vi "PID_controller_05.vi"() -> ()   [LabVIEW 2011]
uses:
  <vilib>/Platform/TimedLoop/XDataNode/nitl_modes.ctl
  <vilib>/Platform/TimedLoop/XDataNode/timing_clust.ctl
  <vilib>/Platform/TimedLoop/XDataNode/wakeup.ctl
  <vilib>/Platform/TimedLoop/XDataNode/XDataNode.xnode
  <vilib>/Platform/TimedLoop/XDataNode/XDNodeRunTimeDep.lvlib
panel:
  out "Numeric":dbl
  out "x-y":dbl
  out "S00":dbl
  out "S10":dbl
  out "S20":dbl
  out "S11":dbl
  out "S01":dbl
  out "weight":dbl[](array[numeric])
  in  "# of points to watch":i32
  in  "alpha":dbl=-1.0
  out "t0":dbl
  out "error(t)":cluster{dbl, "Value":dbl}[](array[cluster])
  out "error out":errorcluster
  out "first":bool=TRUE
  out "P (torr)":string
  out "XY Graph":cluster{dbl, "Value":dbl}[](graph)
  out "current value":dbl
  in  "stop":bool
  in  "Period (s)":dbl
  out "dValue":dbl
  out "derivative":dbl
  out "integral":dbl
  out "error":dbl
  out "Current angle (deg)":dbl
  in  "Kd":dbl
  in  "Ki":dbl
  in  "Kp":dbl
  out "Current P (torr)":dbl
  in  "Set Point (torr)":dbl
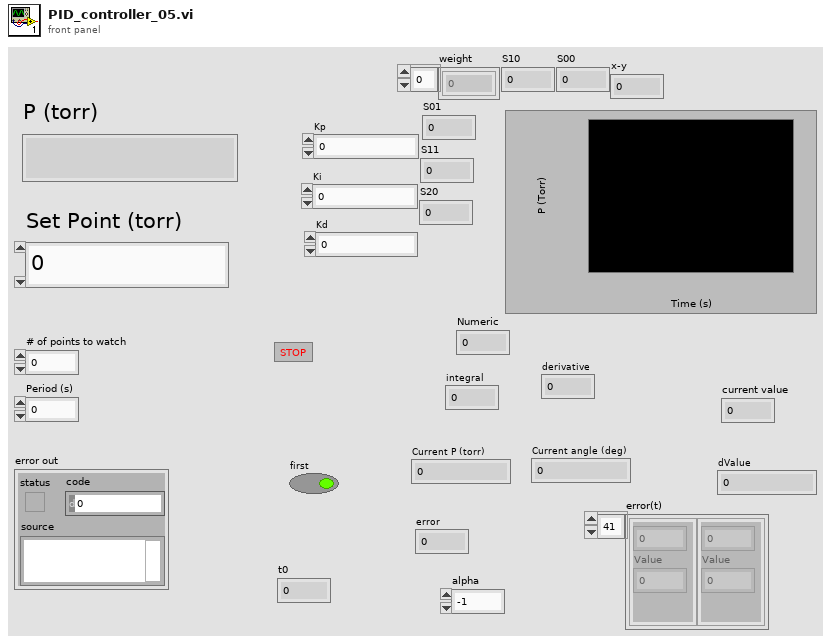
[diagram p1: front panel]
types:
  T1 = typedef "XDNodeRunTimeDep.lvlib/nitl_modes.ctl" = enum32{"No Change", "Process missed periods, maintain original phase", "Discard missed periods, maintain original phase", "Process missed periods, ignore original phase", "Discard missed periods, ignore original phase"}
  T2 = typedef "XDNodeRunTimeDep.lvlib/timing_clust.ctl" = cluster{"Expected End [f-1]":u64, "Actual End [f-1]":u64, "Finished Late? [f-1]":bool, "Expected End [i-1]":u64, "Actual End [i-1]":u64, "Finished Late? [i-1]":bool, "Expected Start [i]":u64, "Actual Start [i]":u64, "Expected Start [f]":u64, "Actual Start [f]":u64, "Source Name":string, "Structure Name":string, "Period":i64, "Deadline":i64, "Offset":i64, "Start":i64, "Priority":i32, "Timeout":i32, "Mode":T1, "Wakeup Reason":T3, "Error":errorcluster, "Source Type":string, "Secondary Source Type":string, "Global End Time":u64, "Global Start Time":u64, "Frame Duration":u64, "Iteration Duration":u64, "Assigned CPU":i32, "I/O Scan Engine Mode":u32}
  T3 = typedef "XDNodeRunTimeDep.lvlib/wakeup.ctl" = enum32{"Normal", "Aborted", "Asynchronous wakeup", "Timing source error", "Timed loop error", "Timeout"}
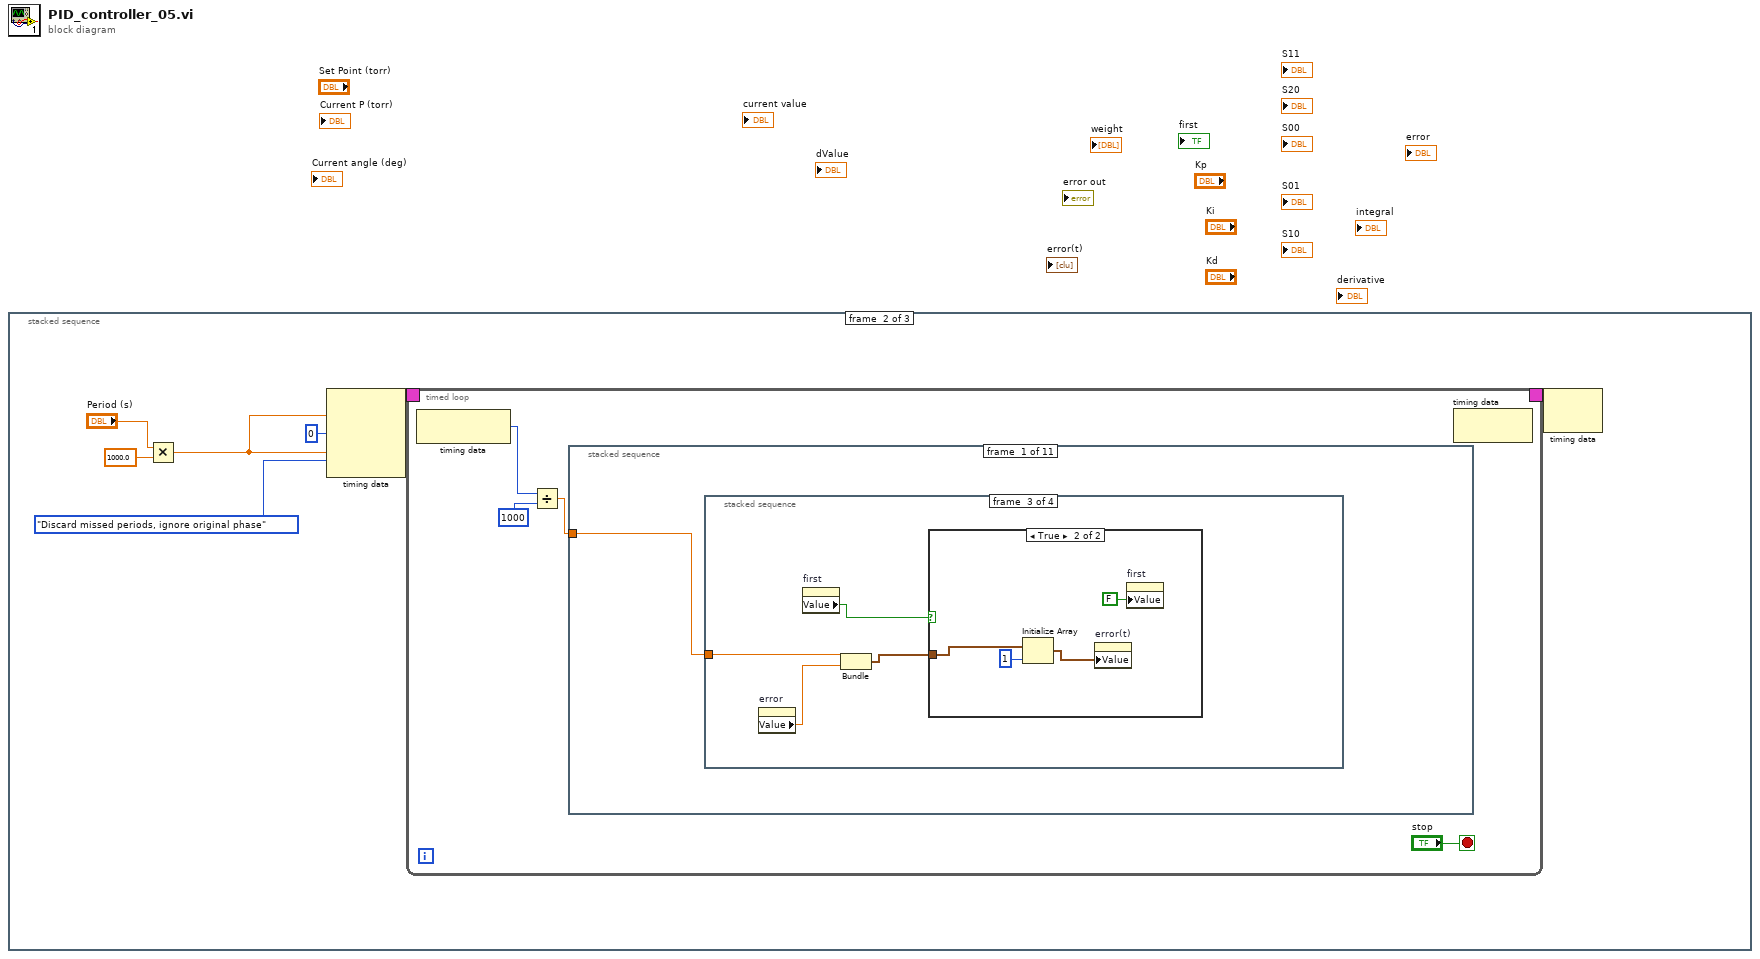
[diagram p0: block diagram]
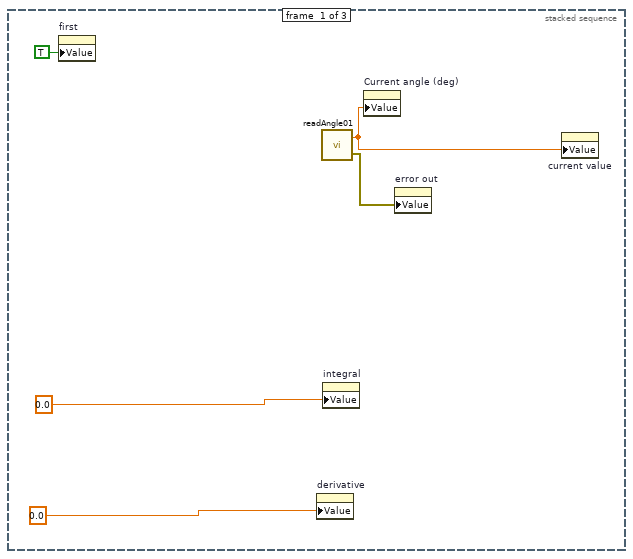
[diagram p2: hidden frame]
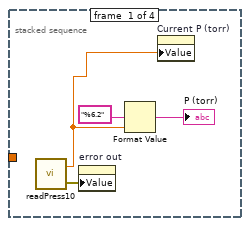
[diagram p3: hidden frame]
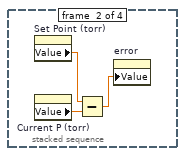
[diagram p4: hidden frame]
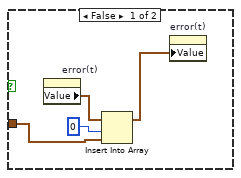
[diagram p5: hidden frame]
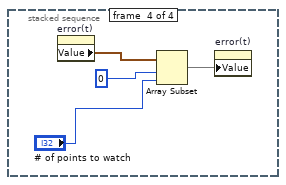
[diagram p6: hidden frame]
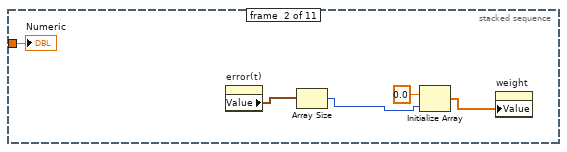
[diagram p7: hidden frame]
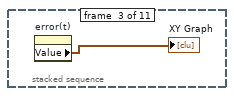
[diagram p8: hidden frame]
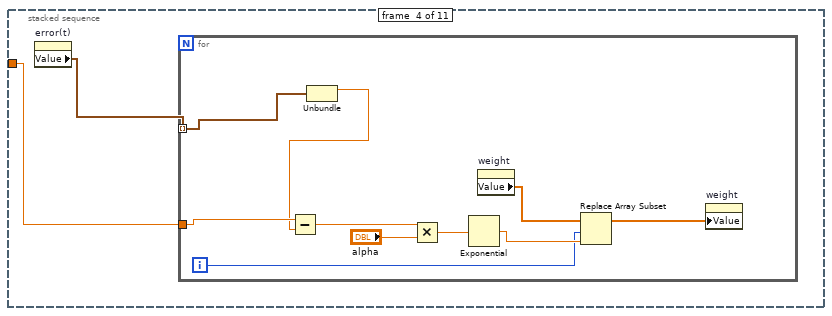
[diagram p9: hidden frame]
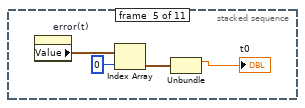
[diagram p10: hidden frame]
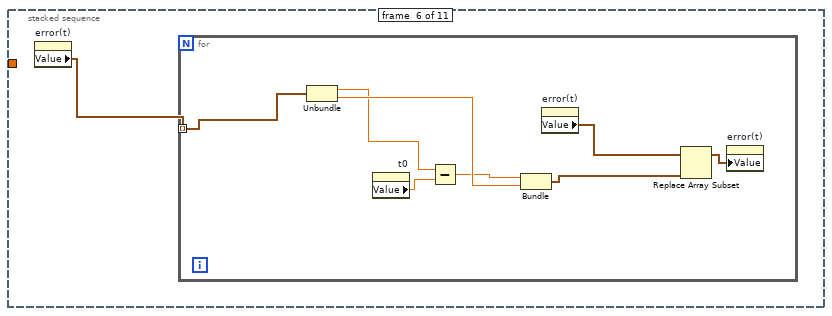
[diagram p11: hidden frame]
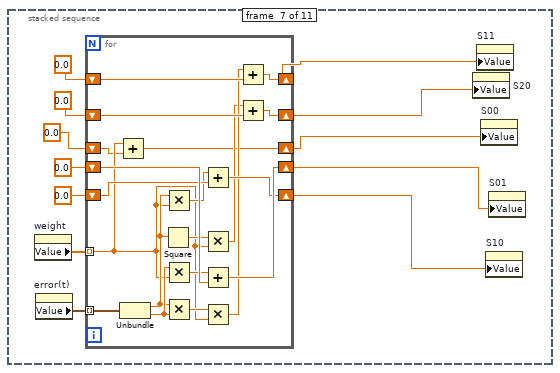
[diagram p12: hidden frame]
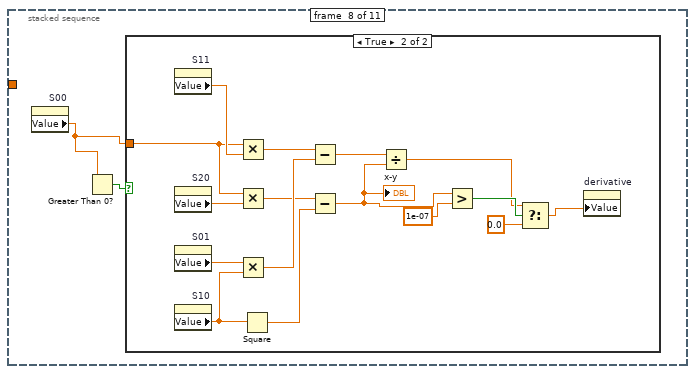
[diagram p13: hidden frame]
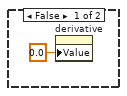
[diagram p14: hidden frame]
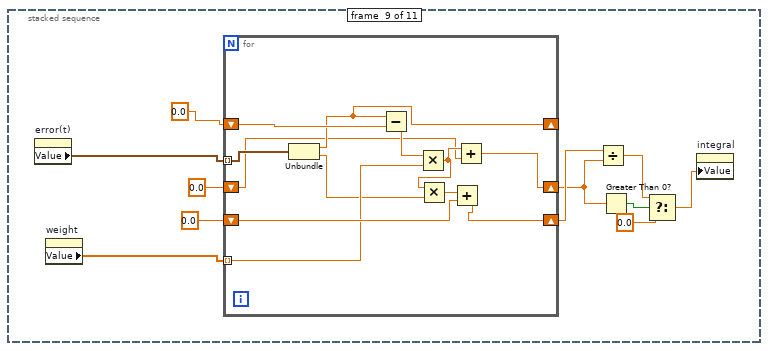
[diagram p15: hidden frame]
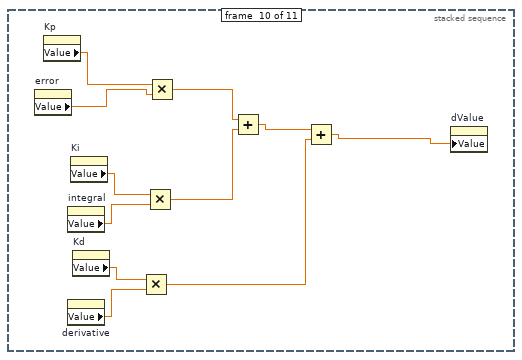
[diagram p16: hidden frame]
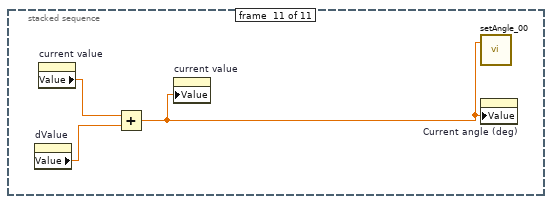
[diagram p17: hidden frame]
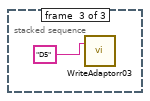
[diagram p18: hidden frame]
diagram:
  n1 = stacked-sequence {
    frame #0 {
      n2 = property on="first" class="Bool (strict)"("Value"=TRUE ("first")) -> ()  [unwired: 2 in, 2 out]
      n3 = property on="derivative" class="DigNum (strict)"("Value"=0.0 ("derivative")) -> ()  [unwired: 2 in, 2 out]
      n4 = call "readAngle01.vi"() -> ("angle"=w1:dbl, "error out"=w2:errorcluster)  [unwired: 1 in]
      n5 = property on="integral" class="DigNum (strict)"("Value"=0.0 ("integral")) -> ()  [unwired: 2 in, 2 out]
      n6 = property on="Current angle (deg)" class="DigNum (strict)"("Value"=w1) -> ()  [unwired: 2 in, 2 out]
      n7 = property on="error out" class="Clust (strict)"("Value"=w2) -> ()  [unwired: 2 in, 2 out]
      n8 = property on="current value" class="DigNum (strict)"("Value"=w1) -> ()  [unwired: 2 in, 2 out]
    }
    frame #1 {
      n9 = Multiply(x="Period (s)", y=1000.0) -> (x*y=w7:dbl)
      n10 = node-c288(w7, i64 0 ("Offset"), w7, nitl_modes."Discard missed periods, ignore original phase" ("Mode")) -> (w12:T2)
      n11 = timed-loop {
        timing: w12 -> [_]
        timing-out: [_] -> w11
        stop <- "stop" stop-if-true
        n12 = node-c288() -> (w13:i64)  [unwired: 1 in]
        n13 = Divide(x=w13, y=i64 1000) -> (x/y=w14:dbl)
        n14 = stacked-sequence {
          tunnel: w14 -> [w17 w41 _ w47 _ _ _ _ _ _ _]
          frame #0 {
            n15 = stacked-sequence {
              tunnel: w17 -> [_ _ w27 _]
              frame #0 {
                n16 = call "readPress10.vi"() -> ("P"=w18:dbl, "error out"=w19:errorcluster)  [unwired: 1 in]
                n17 = property on="error out" class="Clust (strict)"("Value"=w19) -> ()  [unwired: 2 in, 2 out]
                n18 = Format Value(format string="%6.2", value (0)=w18) -> (output string=→"P (torr)":string)  [unwired: 1 in]
                n19 = property on="Current P (torr)" class="DigNum (strict)"("Value"=w18) -> ()  [unwired: 2 in, 2 out]
              }
              frame #1 {
                n20 = property on="Set Point (torr)" class="DigNum (strict)"() -> ("Value"=w23:dbl)  [unwired: 2 in, 2 out]
                n21 = property on="Current P (torr)" class="DigNum (strict)"() -> ("Value"=w24:dbl)  [unwired: 2 in, 2 out]
                n22 = Subtract(x=w23, y=w24) -> (x-y=w22:dbl)
                n23 = property on="error" class="DigNum (strict)"("Value"=w22) -> ()  [unwired: 2 in, 2 out]
              }
              frame #2 {
                n24 = property on="error" class="DigNum (strict)"() -> ("Value"=w26:dbl)  [unwired: 2 in, 2 out]
                n25 = property on="first" class="Bool (strict)"() -> ("Value"=w28:bool)  [unwired: 2 in, 2 out]
                n26 = Bundle(w27, "Value"=w26) -> (w25:cluster{dbl, "Value":dbl})  [unwired: 1 in]
                n27 = case shown="True" w28 {
                  tunnel: w25 -> [w30 w35]
                  frame False {
                    n28 = property on="error(t)" class="Arr (strict)"() -> ("Value"=w31:cluster{dbl, "Value":dbl}[])  [unwired: 2 in, 2 out]
                    n29 = Insert Into Array(array=w31, index=0, new element=w30) -> (w29:cluster{dbl, "Value":dbl}[])
                    n30 = property on="error(t)" class="Arr (strict)"("Value"=w29) -> ()  [unwired: 2 in, 2 out]
                  }
                  frame True {
                    n31 = Initialize Array(w35, 1 ("dimension size")) -> (w33:cluster{dbl, "Value":dbl}[])
                    n32 = property on="error(t)" class="Arr (strict)"("Value"=w33) -> ()  [unwired: 2 in, 2 out]
                    n33 = property on="first" class="Bool (strict)"("Value"=FALSE ("first")) -> ()  [unwired: 2 in, 2 out]
                  }
                }
              }
              frame #3 {
                n34 = property on="error(t)" class="Arr (strict)"() -> ("Value"=w38:cluster{dbl, "Value":dbl}[])  [unwired: 2 in, 2 out]
                n35 = Array Subset(array=w38, index=0, length="# of points to watch") -> (w40:cluster{dbl, "Value":dbl}[])
                n36 = property on="error(t)" class="Arr (strict)"("Value"=w40) -> ()  [unwired: 2 in, 2 out]
              }
            }
          }
          frame #1 {
            n37 = property on="error(t)" class="Arr (strict)"() -> ("Value"=w45:cluster{dbl, "Value":dbl}[])  [unwired: 2 in, 2 out]
            n38 = Array Size(array=w45) -> (size(s)=w43:i32)
            n39 = Initialize Array(0.0 ("element"), w43) -> (w42:dbl[])
            n40 = property on="weight" class="Arr (strict)"("Value"=w42) -> ()  [unwired: 2 in, 2 out]
            "Numeric" <- w41
          }
          frame #2 {
            n41 = property on="error(t)" class="Arr (strict)"() -> ("Value"=→"XY Graph":cluster{dbl, "Value":dbl}[])  [unwired: 2 in, 2 out]
          }
          frame #3 {
            n42 = property on="error(t)" class="Arr (strict)"() -> ("Value"=w48:cluster{dbl, "Value":dbl}[])  [unwired: 2 in, 2 out]
            n43 = for {
              tunnel: w48 -> [w58] mode=indexing
              tunnel: w47 -> [w55]
              i -> [w50]
              n44 = Unbundle(w58) -> (w54:dbl)  [unwired: 1 out]
              n45 = Subtract(x=w55, y=w54) -> (x-y=w53:dbl)
              n46 = Multiply(x=w53, y="alpha") -> (x*y=w56:dbl)
              n47 = Exponential(1:w56) -> (0:w52:dbl)
              n48 = property on="weight" class="Arr (strict)"() -> ("Value"=w51:dbl[])  [unwired: 2 in, 2 out]
              n49 = Replace Array Subset(array=w51, new element=w52, index=w50) -> (w49:dbl[])
              n50 = property on="weight" class="Arr (strict)"("Value"=w49) -> ()  [unwired: 2 in, 2 out]
            }
          }
          frame #4 {
            n51 = property on="error(t)" class="Arr (strict)"() -> ("Value"=w62:cluster{dbl, "Value":dbl}[])  [unwired: 2 in, 2 out]
            n52 = Index Array(array=w62, index=0) -> (element=w60:cluster{dbl, "Value":dbl})
            n53 = Unbundle(w60) -> (→"t0":dbl)  [unwired: 1 out]
          }
          frame #5 {
            n54 = property on="error(t)" class="Arr (strict)"() -> ("Value"=w63:cluster{dbl, "Value":dbl}[])  [unwired: 2 in, 2 out]
            n55 = for {
              tunnel: w63 -> [w68] mode=indexing
              n56 = Unbundle(w68) -> (w65:dbl, "Value"=w70:dbl)
              n57 = property on="t0" class="DigNum (strict)"() -> ("Value"=w71:dbl)  [unwired: 2 in, 2 out]
              n58 = Subtract(x=w65, y=w71) -> (x-y=w66:dbl)
              n59 = Bundle(w66, "Value"=w70) -> (w64:cluster{dbl, "Value":dbl})  [unwired: 1 in]
              n60 = property on="error(t)" class="Arr (strict)"() -> ("Value"=w69:cluster{dbl, "Value":dbl}[])  [unwired: 2 in, 2 out]
              n61 = Replace Array Subset(array=w69, new element=w64) -> (w67:cluster{dbl, "Value":dbl}[])  [unwired: 1 in]
              n62 = property on="error(t)" class="Arr (strict)"("Value"=w67) -> ()  [unwired: 2 in, 2 out]
            }
          }
          frame #6 {
            n63 = property on="weight" class="Arr (strict)"() -> ("Value"=w78:dbl[])  [unwired: 2 in, 2 out]
            n64 = property on="error(t)" class="Arr (strict)"() -> ("Value"=w83:cluster{dbl, "Value":dbl}[])  [unwired: 2 in, 2 out]
            n65 = for {
              tunnel: w83 -> [w99] mode=indexing
              shift-right: [w100] -> w73
              shift-left: 0.0 -> [w103]
              shift-right: [w96] -> w76
              shift-left: 0.0 -> [w102]
              shift-right: [w95] -> w75
              shift-left: 0.0 -> [w101]
              shift-right: [w97] -> w72
              shift-left: 0.0 -> [w98]
              tunnel: w78 -> [w86] mode=indexing
              shift-right: [w84] -> w74
              shift-left: 0.0 -> [w85]
              n66 = Add(x=w86, y=w85) -> (x+y=w84:dbl)
              n67 = Unbundle(w99) -> (w88:dbl, "Value"=w94:dbl)
              n68 = Square(x=w88) -> (x^2=w90:dbl)
              n69 = Multiply(x=w88, y=w86) -> (x*y=w87:dbl)
              n70 = Multiply(x=w94, y=w86) -> (x*y=w93:dbl)
              n71 = Multiply(x=w88, y=w94) -> (x*y=w92:dbl)
              n72 = Add(x=w87, y=w98) -> (x+y=w97:dbl)
              n73 = Multiply(x=w90, y=w86) -> (x*y=w89:dbl)
              n74 = Add(x=w93, y=w103) -> (x+y=w100:dbl)
              n75 = Multiply(x=w92, y=w86) -> (x*y=w91:dbl)
              n76 = Add(x=w91, y=w102) -> (x+y=w96:dbl)
              n77 = Add(x=w89, y=w101) -> (x+y=w95:dbl)
            }
            n78 = property on="S20" class="DigNum (strict)"("Value"=w75) -> ()  [unwired: 2 in, 2 out]
            n79 = property on="S11" class="DigNum (strict)"("Value"=w76) -> ()  [unwired: 2 in, 2 out]
            n80 = property on="S00" class="DigNum (strict)"("Value"=w74) -> ()  [unwired: 2 in, 2 out]
            n81 = property on="S10" class="DigNum (strict)"("Value"=w72) -> ()  [unwired: 2 in, 2 out]
            n82 = property on="S01" class="DigNum (strict)"("Value"=w73) -> ()  [unwired: 2 in, 2 out]
          }
          frame #7 {
            n83 = property on="S00" class="DigNum (strict)"() -> ("Value"=w104:dbl)  [unwired: 2 in, 2 out]
            n84 = Greater Than 0?(x=w104) -> (x > 0?=w105:bool)
            n85 = case shown="True" w105 {
              tunnel: w104 -> [_ w114]
              frame False {
                n86 = property on="derivative" class="DigNum (strict)"("Value"=0.0 ("derivative")) -> ()  [unwired: 2 in, 2 out]
              }
              frame True {
                n87 = property on="S11" class="DigNum (strict)"() -> ("Value"=w116:dbl)  [unwired: 2 in, 2 out]
                n88 = property on="S20" class="DigNum (strict)"() -> ("Value"=w115:dbl)  [unwired: 2 in, 2 out]
                n89 = property on="S01" class="DigNum (strict)"() -> ("Value"=w113:dbl)  [unwired: 2 in, 2 out]
                n90 = property on="S10" class="DigNum (strict)"() -> ("Value"=w117:dbl)  [unwired: 2 in, 2 out]
                n91 = Multiply(x=w114, y=w116) -> (x*y=w122:dbl)
                n92 = Multiply(x=w114, y=w115) -> (x*y=w120:dbl)
                n93 = Multiply(x=w113, y=w117) -> (x*y=w121:dbl)
                n94 = Square(x=w117) -> (x^2=w119:dbl)
                n95 = Subtract(x=w122, y=w121) -> (x-y=w118:dbl)
                n96 = Subtract(x=w120, y=w119) -> (x-y=w112:dbl)
                "x-y" <- w112
                n97 = Divide(x=w118, y=w112) -> (x/y=w108:dbl)
                n98 = Greater?(x=w112, y=1e-07) -> (0:w110:bool)
                n99 = Select(t=w108, s=w110, f=0.0) -> (s? t:f=w109:dbl)
                n100 = property on="derivative" class="DigNum (strict)"("Value"=w109) -> ()  [unwired: 2 in, 2 out]
              }
            }
          }
          frame #8 {
            n101 = property on="error(t)" class="Arr (strict)"() -> ("Value"=w133:cluster{dbl, "Value":dbl}[])  [unwired: 2 in, 2 out]
            n102 = property on="weight" class="Arr (strict)"() -> ("Value"=w131:dbl[])  [unwired: 2 in, 2 out]
            n103 = for {
              tunnel: w133 -> [w145] mode=indexing
              shift-right: [w143] -> _
              shift-left: 0.0 -> [w144]
              tunnel: w131 -> [w138] mode=indexing
              shift-right: [w139] -> w128
              shift-left: 0.0 -> [w140]
              shift-right: [w135] -> w127
              shift-left: 0.0 -> [w134]
              n104 = Unbundle(w145) -> (w143:dbl, "Value"=w137:dbl)
              n105 = Subtract(x=w143, y=w144) -> (x-y=w142:dbl)
              n106 = Multiply(x=w142, y=w138) -> (x*y=w136:dbl)
              n107 = Multiply(x=w136, y=w137) -> (x*y=w141:dbl)
              n108 = Add(x=w141, y=w140) -> (x+y=w139:dbl)
              n109 = Add(x=w136, y=w134) -> (x+y=w135:dbl)
            }
            n110 = Divide(x=w128, y=w127) -> (x/y=w125:dbl)
            n111 = Greater Than 0?(x=w127) -> (x > 0?=w126:bool)
            n112 = Select(t=w125, s=w126, f=0.0) -> (s? t:f=w123:dbl)
            n113 = property on="integral" class="DigNum (strict)"("Value"=w123) -> ()  [unwired: 2 in, 2 out]
          }
          frame #9 {
            n114 = property on="error" class="DigNum (strict)"() -> ("Value"=w156:dbl)  [unwired: 2 in, 2 out]
            n115 = property on="Kp" class="DigNum (strict)"() -> ("Value"=w155:dbl)  [unwired: 2 in, 2 out]
            n116 = property on="integral" class="DigNum (strict)"() -> ("Value"=w153:dbl)  [unwired: 2 in, 2 out]
            n117 = property on="derivative" class="DigNum (strict)"() -> ("Value"=w151:dbl)  [unwired: 2 in, 2 out]
            n118 = property on="Ki" class="DigNum (strict)"() -> ("Value"=w154:dbl)  [unwired: 2 in, 2 out]
            n119 = property on="Kd" class="DigNum (strict)"() -> ("Value"=w152:dbl)  [unwired: 2 in, 2 out]
            n120 = Multiply(x=w152, y=w151) -> (x*y=w148:dbl)
            n121 = Multiply(x=w154, y=w153) -> (x*y=w149:dbl)
            n122 = Multiply(x=w155, y=w156) -> (x*y=w150:dbl)
            n123 = Add(x=w150, y=w149) -> (x+y=w147:dbl)
            n124 = Add(x=w147, y=w148) -> (x+y=w146:dbl)
            n125 = property on="dValue" class="DigNum (strict)"("Value"=w146) -> ()  [unwired: 2 in, 2 out]
          }
          frame #10 {
            n126 = property on="dValue" class="DigNum (strict)"() -> ("Value"=w158:dbl)  [unwired: 2 in, 2 out]
            n127 = property on="current value" class="DigNum (strict)"() -> ("Value"=w159:dbl)  [unwired: 2 in, 2 out]
            n128 = Add(x=w159, y=w158) -> (x+y=w157:dbl)
            n129 = property on="current value" class="DigNum (strict)"("Value"=w157) -> ()  [unwired: 2 in, 2 out]
            n130 = call "setAngle_00.vi"("Angle (deg)"=w157) -> ()  [unwired: 1 in, 1 out]
            n131 = property on="Current angle (deg)" class="DigNum (strict)"("Value"=w157) -> ()  [unwired: 2 in, 2 out]
          }
        }
        n132 = node-c288() -> ()  [unwired: 1 in, 1 out]
      }
      n133 = node-c288(w11) -> ()  [unwired: 1 out]
    }
    frame #2 {
      n134 = call "WriteAdaptorr03.vi"("string to write"="D5") -> ()  [unwired: 1 in, 1 out]
    }
  }
